vi "Get Events.vi"(11 "Hot And Cold Source Unit View in":refnum<class "Hot And Cold Source Unit View.lvclass">) -> (2 "Events":T1, 3 "Hot And Cold Source Unit View out":refnum<class "Hot And Cold Source Unit View.lvclass">)   [LabVIEW 2013, in "Hot And Cold Source Unit View.lvlib" / "Hot And Cold Source Unit View.lvclass"]
uses:
  Hot And Cold Source Unit View.lvclass
  Typedef/Events.ctl
  Hot And Cold Source Unit View.lvclass/Hot And Cold Source Unit View.ctl
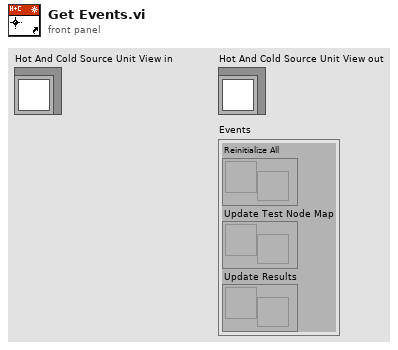
[diagram p1: front panel]
types:
  T1 = typedef "Hot And Cold Source Unit View.lvlib/Hot And Cold Source Unit View.lvclass/Events.ctl" = cluster{"Reinitialize All":refnum<user-event>, "Update Test Node Map":refnum<user-event>, "Update Results":refnum<user-event>}
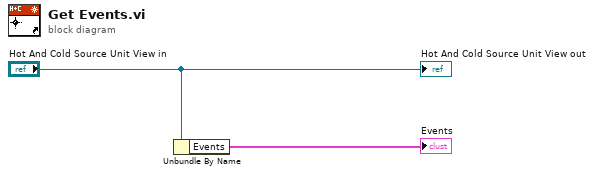
[diagram p0: block diagram]
diagram:
  n1 = Unbundle By Name("Hot And Cold Source Unit View in") -> ("Events"=→"Events":T1)
  "Hot And Cold Source Unit View out" <- "Hot And Cold Source Unit View in"
